vi "NewColour selection.vi"(1 "Defined Colour":u32(colorbox), 2 "Default Colour":u32(colorbox), 3 "Old Color":u32(colorbox)) -> (0 "New Colour":u32(colorbox))   [LabVIEW 2012, in "ColourUpStructures.lvlib"]
doc: "Compare Old Colour with Default and Defined colour. <b>New Colour</b> will be more fare away from Default or Defined Colour."
uses:
  ColourUpStructures.lvlib
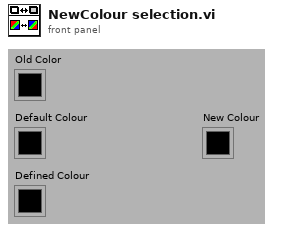
[diagram p1: front panel]
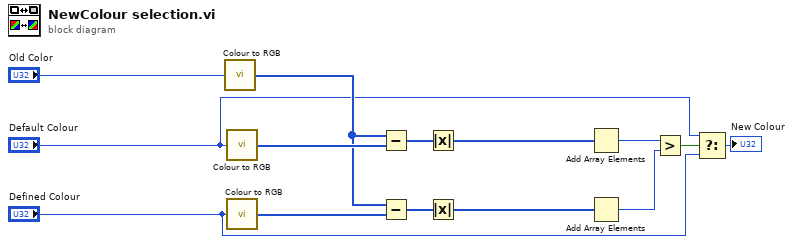
[diagram p0: block diagram]
diagram:
  n1 = call "Colour to RGB.vi"("Colour"="Old Color") -> ("Colours[R,G,B]"=w4:u8[])  [unwired: 14 in]
  n2 = call "Colour to RGB.vi"("Colour"="Default Colour") -> ("Colours[R,G,B]"=w8:u8[])  [unwired: 14 in]
  n3 = call "Colour to RGB.vi"("Colour"="Defined Colour") -> ("Colours[R,G,B]"=w3:u8[])  [unwired: 14 in]
  n4 = Subtract(x=w4, y=w8) -> (x-y=w14:i16[])
  n5 = Subtract(x=w4, y=w3) -> (x-y=w13:i16[])
  n6 = Absolute Value(x=w14) -> (abs(x)=w6:i16[])
  n7 = Absolute Value(x=w13) -> (abs(x)=w7:i16[])
  n8 = Add Array Elements(numeric array=w6) -> (sum=w12:i16)
  n9 = Add Array Elements(numeric array=w7) -> (sum=w11:i16)
  n10 = Greater?(x=w12, y=w11) -> (0:w10:bool)
  n11 = Select(t="Default Colour", s=w10, f="Defined Colour") -> (s? t:f=→"New Colour":u32)
